vi "Disable Property.vi"() -> ()   [LabVIEW 2021]
panel:
  in  "Disabled":T1(ring)
  in  "Indicator":dbl
  in  "stop":bool
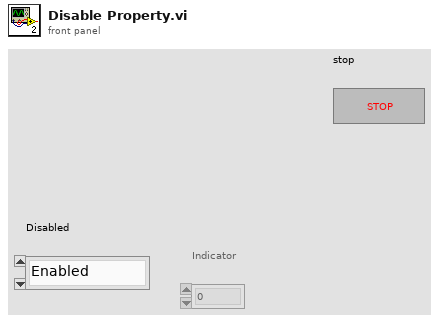
[diagram p1: front panel]
types:
  T1 = enum8{"Enabled", "Disabled", "Disabled and Grayed Out"}
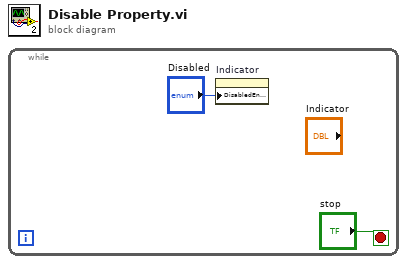
[diagram p0: block diagram]
diagram:
  n1 = while {
    stop <- "stop" stop-if-true
    n2 = property on="Indicator" class="DigNum (strict)"("DisabledEnum"="Disabled") -> ()  [unwired: 2 in, 2 out]
  }
